vi "BRig_dataExp_I_trialUntilReward.vi"() -> (2 "output_I_trialUntilReward":i32)   [LabVIEW 2014]
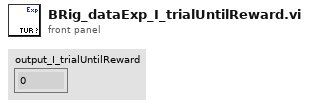
[diagram p1: front panel]
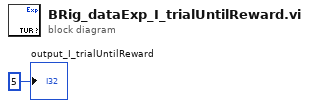
[diagram p0: block diagram]
diagram:
  "output_I_trialUntilReward" <- 5 ("output_iBlock")
